vi "Reset.vi"(8 "error in (no error)":errorcluster, 11 "Serial Controller in":refnum<class "Serial Controller.lvclass">) -> (0 "error out":errorcluster, 3 "Serial Controller out":refnum<class "Serial Controller.lvclass">)   [LabVIEW 2013, in "Serial Controller.lvclass"]
uses:
  Serial Controller.lvclass
  Serial Controller.lvclass/Serial Controller.ctl
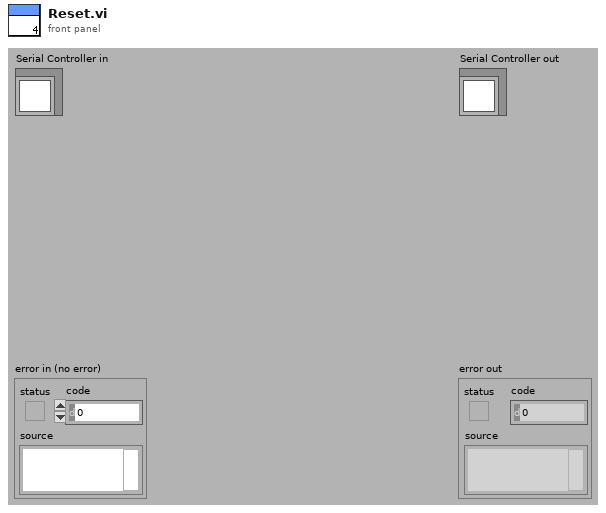
[diagram p1: front panel]
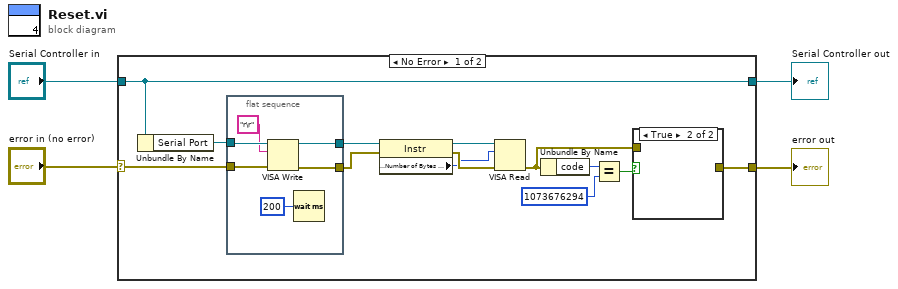
[diagram p0: block diagram]
diagram:
  n1 = case shown="No Error" "error in (no error)" {
    selector: "error in (no error)" -> [w17 w26]
    tunnel: [w5 w26] -> w3
    tunnel: [w16 w25] -> w1
    tunnel: "Serial Controller in" -> [w16 w25]
    frame No Error {
      n2 = Unbundle By Name(w16) -> ("Serial Port"=w15:refnum<visa-resource-name>)
      n3 = flat-sequence {
        tunnel: w17 -> [w23]
        tunnel: [w21] -> w12
        tunnel: w15 -> [w22]
        tunnel: [w19] -> w14
        frame #0 {
          n4 = VISA Write(VISA resource name=w22, write buffer="r\r", error in (no error)=w23) -> (VISA resource name out=w19:refnum<visa-resource-name>, error out=w21:errorcluster)  [unwired: 1 out]
          n5 = Wait (ms)(milliseconds to wait=u32 200) -> ()  [unwired: 1 out]
        }
      }
      n6 = property class="Instr"(reference=w14, error in=w12) -> (reference out=w13:refnum<visa-resource-name>, error out=w11:errorcluster, "Serial Settings:Number of Bytes at Serial Port"=w10:u32)
      n7 = VISA Read(VISA resource name=w13, byte count=w10, error in (no error)=w11) -> (error out=w6:errorcluster)  [unwired: 3 out]
      n8 = Unbundle By Name(w6) -> ("code"=w9:i32)
      n9 = Equal?(x=w9, y=1073676294) -> (x = y?=w7:bool)
      n10 = case shown="True" w7 {
        tunnel: w6 -> [w18 _]
        tunnel: [w18 _] -> w5
        frame False {
        }
        frame True {
        }
      }
    }
    frame Error {
    }
  }
  "error out" <- w3
  "Serial Controller out" <- w1
